vi "niScope Configure Horizontal Timing.vi"(0 "instrument handle":refnum<k15>, 1 "number of records":i32=1, 2 "enforce realtime":bool=TRUE, 5 "min sample rate":dbl=20000000.0 format="%^.2e", 9 "reference position":dbl=50.0 format="%.1f", 11 "error in":errorcluster, 12 "min record length":i32=1000) -> (4 "instrument handle out":refnum<k15>, 15 "error out":errorcluster)   [LabVIEW 2013]
doc: "Configures the common properties of the horizontal subsystem for a single record or multirecord acquisition, such as minimum sample rate and acquisition size."
uses:
  niScope_32.dll
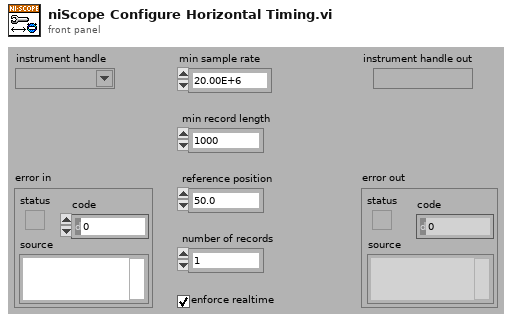
[diagram p1: front panel]
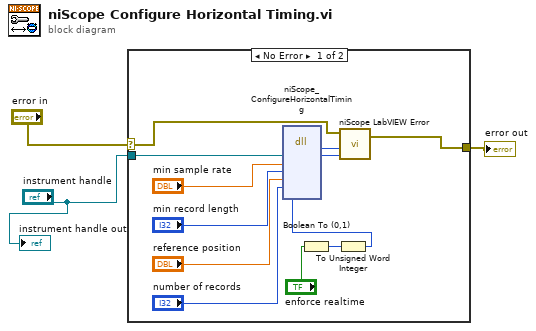
[diagram p0: block diagram]
diagram:
  n1 = case shown="No Error" "error in" {
    selector: "error in" -> [w4 w16]
    tunnel: [w8 w16] -> w3
    tunnel: "instrument handle" -> [w15 _]
    frame No Error {
      n2 = Boolean To (0,1)(Boolean="enforce realtime") -> (0, 1=w6:i16)
      n3 = To Unsigned Word Integer(number=w6) -> (unsigned 16bit integer=w5:u16)
      n4 = dll-call lib="niScope_*.*" fn="niScope_ConfigureHorizontalTiming"("instrument handle"=w15, "minSampleRate"="min sample rate", "minNumPts"="min record length", "refPosition"="reference position", "numRecords"="number of records", "enforceRealtime"=w5) -> ("status"=w10:i32, "instrument handle"=w9:u32)  [unwired: 8 in, 2 out]
      n5 = call "niScope LabVIEW Error.vi"("instrument handle"=w9, "niScope error code (0)"=w10, "error in (no error)"=w4) -> ("error out"=w8:errorcluster)  [unwired: 2 in]
    }
    frame Error {
    }
  }
  "error out" <- w3
  "instrument handle out" <- "instrument handle"
